vi "Test.vi"() -> ()   [LabVIEW 2017]
uses:
  <vilib>/Skyline/Tag/Shared/typedefs/DataType.ctl
  <vilib>/Skyline/Tag/Wrapper/Wrapper AMQP_class/Open Tag AMQP.vi
  <vilib>/Skyline/Tag/Wrapper/Wrapper_class/Read Tag (DBL).vi
  <vilib>/Skyline/Tag/Wrapper/Wrapper_class/Close Tag (Single).vi
  <vilib>/Skyline/Tag/Wrapper/Wrapper_class/NI Skyline Tag.lvclass
  <vilib>/Skyline/Tag/Shared/NI Skyline Tag.lvlib
  <vilib>/Skyline/Tag/Wrapper/Wrapper AMQP_class/NI Skyline Tag AMQP.lvclass
panel:
  out "Numeric":i32
  in  "stop":bool
  out "error out":errorcluster
  out "value":dbl
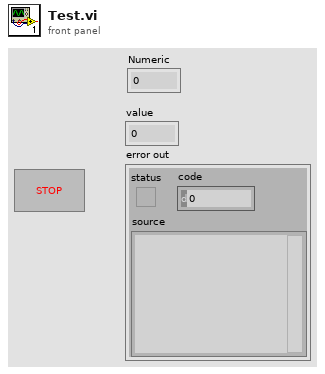
[diagram p1: front panel]
types:
  T1 = typedef "NI Skyline Tag.lvlib/DataType.ctl" = enum32{"Double", "Integer", "String", "Boolean"}
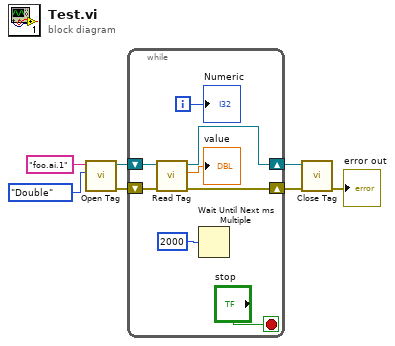
[diagram p0: block diagram]
diagram:
  n1 = call-poly <vilib>:"Open Tag.vi"("data type"=DataType."Double", "path"="foo.ai.1") -> ("error out"=w6:errorcluster, "tag out"=w7:refnum<class "NI Skyline Tag.lvclass">)  [unwired: 8 in]
  n2 = while {
    shift-right: [w12] -> w2
    shift-left: w7 -> [w15]
    shift-right: [w13] -> w3
    shift-left: w6 -> [w14]
    i -> [w8]
    stop <- "stop" stop-if-true
    n3 = call-poly <vilib>:"Read Tag.vi"("error in (no error)"=w14, "tag in"=w15) -> ("error out"=w13:errorcluster, "value"=→"value":dbl, "tag out"=w12:refnum<class "NI Skyline Tag.lvclass">)  [unwired: 5 in, 2 out]
    n4 = Wait Until Next ms Multiple(millisecond multiple=u32 2000) -> ()  [unwired: 1 out]
    "Numeric" <- w8
  }
  n5 = call-poly <vilib>:"Close Tag.vi"("error in (no error)"=w3, "tag in"=w2) -> ("error out"=→"error out":errorcluster)  [unwired: 9 in]
